vi "LoadInterfSetup.vi"(7 "BaseDataPath":path, 8 "ErrIn (NoErr)":errorcluster caption="entrée d'erreur (pas d'erreur)", 9 "IncrSession":bool=TRUE, 10 "LoadIntf?":bool=TRUE, 11 "Interface":path) -> (0 "error out":errorcluster caption="sortie d'erreur", 1 "Experiment Path":path, 2 "Session":i32, 3 "Interface en sortie":refnum<class "Interface.lvclass"> caption="DNL_LabVIEW Object out")   [LabVIEW 2012, in "Interface.lvclass"]
uses:
  Interface.lvclass
  Interface.lvclass/Interface.ctl
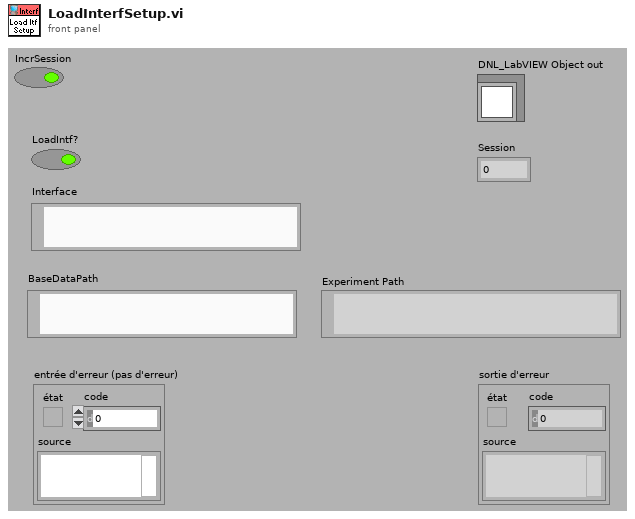
[diagram p1: front panel]
types:
  T1 = typedef "Interface.lvclass/CurveSetup.ctl" = cluster{"CurveName":string, "YParam":string, "XParam":string, "ZParam ":string, "GroupName":string, "LinWdth":u8, "PntCol":u32, "LinCol":u32, "LablFor":u8, "XScale":u32, "YScale":u32, "Interpol":u8, "DisplayName":string, "FillType":i16, "LineStyle":u8, "PntStyle":u8, "BarTyp":u8, "GraphIndex":i32, "Visible":bool, "XScaleName":string, "YScaleName":string, "XYGraph_Ref":refnum<vi>, "Data Only":bool, "DataQ Ref":refnum<queue>, "XParQ Ref":refnum<queue>, "XParamInd":i32, "ScanInd":i32}
  T2 = typedef "2DGraphSetup.ctl" = cluster{"ZDataIndex":i32, "XParIndex":i32, "YParIndex":i32, "FillLineFirst":bool}
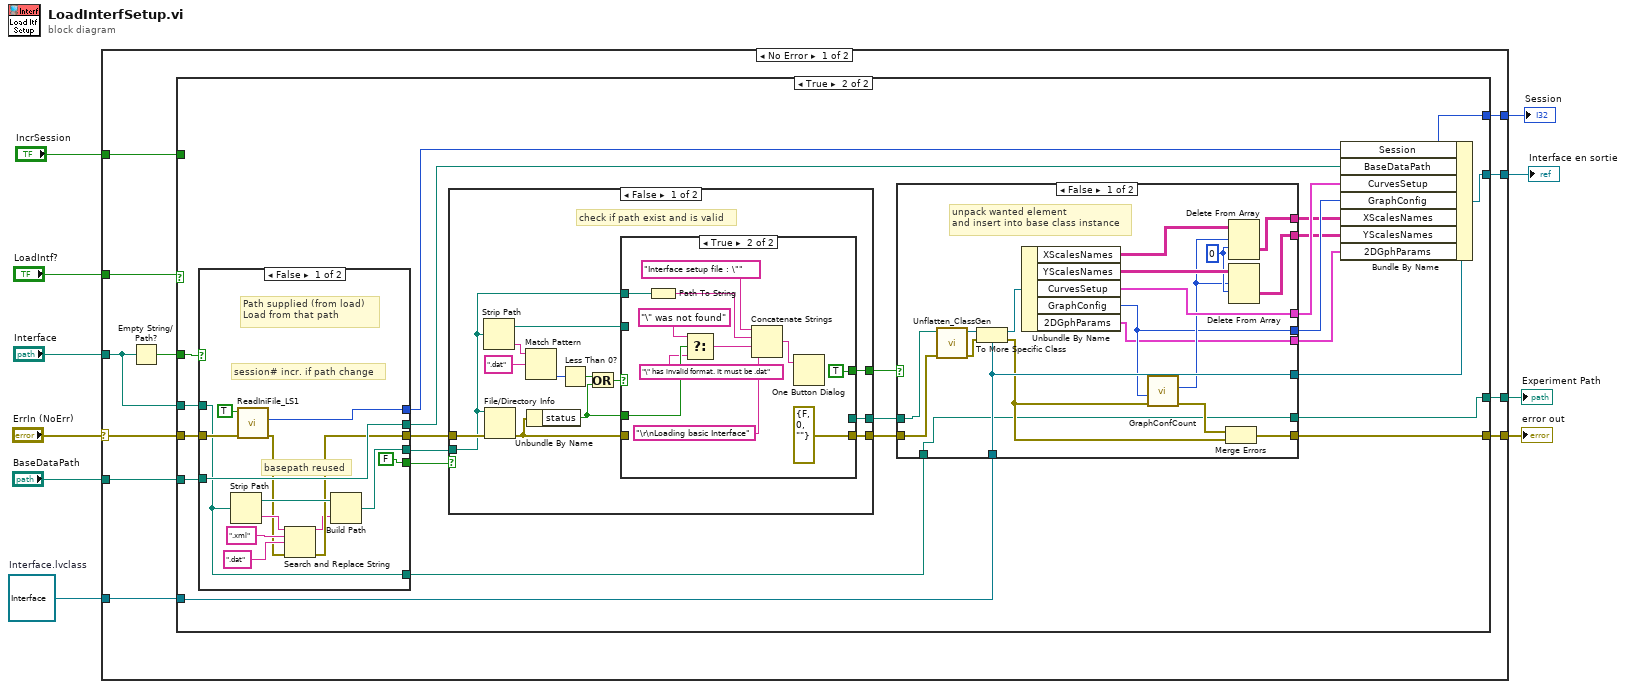
[diagram p0: block diagram]
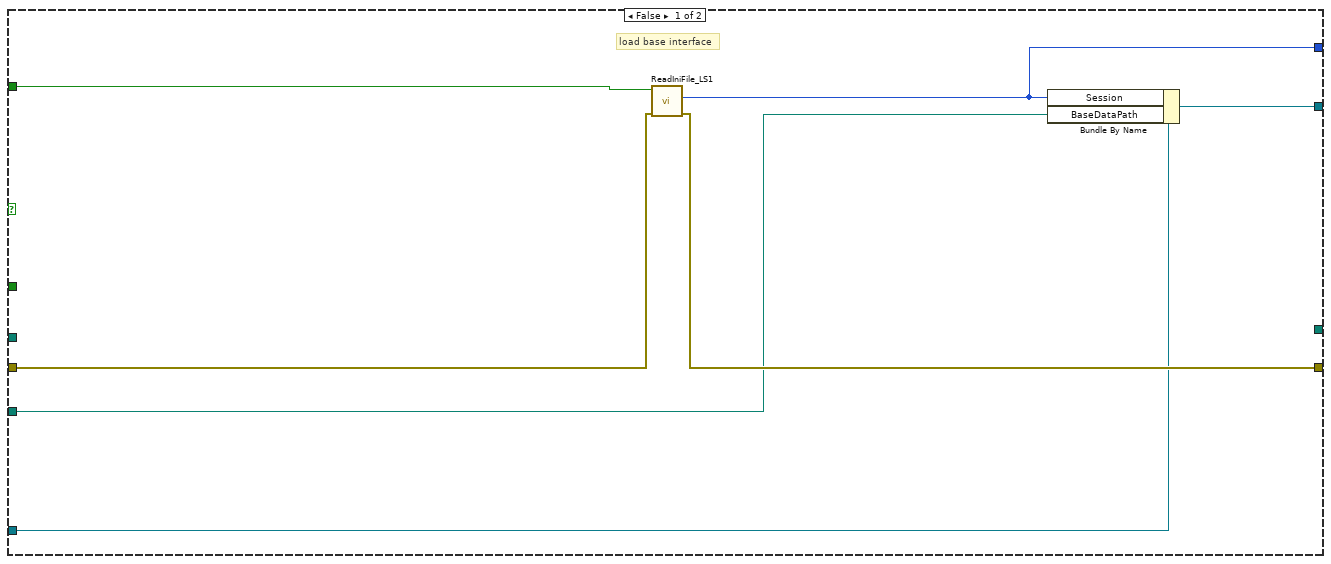
[diagram p2: hidden frame]
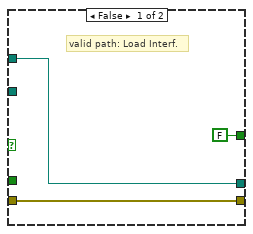
[diagram p3: hidden frame]
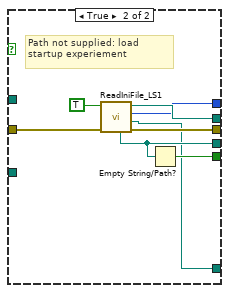
[diagram p5: hidden frame]
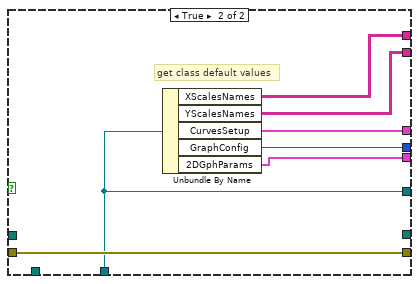
[diagram p6: hidden frame]
diagram:
  w4 = refnum<class "Interface.lvclass"> refnum  # Interface.lvclass
  n1 = case shown="No Error" "ErrIn (NoErr)" {
    selector: "ErrIn (NoErr)" -> [w20 w131]
    tunnel: [w19 w131] -> w9
    tunnel: [w18 w130] -> w8
    tunnel: w4 -> [w21 w130]
    tunnel: "LoadIntf?" -> [w17 _]
    tunnel: "Interface" -> [w15 _]
    tunnel: "BaseDataPath" -> [w14 _]
    tunnel: [w13 _] -> w3
    tunnel: "IncrSession" -> [w12 _]
    tunnel: [w11 _] -> w1
    frame No Error {
      n2 = Empty String/Path?(string/path=w15) -> (empty?=w16:bool)
      n3 = case shown="True" w17 {
        tunnel: w21 -> [w26 w38]
        tunnel: w20 -> [w28 w50]
        tunnel: [w27 w49] -> w19
        tunnel: [w25 w51] -> w18
        tunnel: w16 -> [_ w48]
        tunnel: w15 -> [_ w44]
        tunnel: w14 -> [w24 w39]
        tunnel: [w23 w31] -> w13
        tunnel: w12 -> [w22 _]
        tunnel: [_ w30] -> w11
        frame False {
          # "load base interface"
          n4 = call "ReadIniFile_LS1.vi"("Error in"=w28, "UpdateSess"=w22) -> ("Error out"=w27:errorcluster, "Session"=w23:i32)  [unwired: 4 in, 4 out]
          n5 = Bundle By Name(cluster=w26, "Session"=w23, "BaseDataPath"=w24) -> (w25:refnum<class "Interface.lvclass">)
        }
        frame True {
          n6 = case shown="False" w48 {
            tunnel: w50 -> [w94 w103]
            tunnel: [w91 w102] -> w40
            tunnel: [w92 w101] -> w31
            tunnel: [w84 w100] -> w45
            tunnel: [w82 w97] -> w46
            tunnel: [FALSE w99] -> w47
            tunnel: w44 -> [w90 _]
            tunnel: w39 -> [w91 _]
            tunnel: [w90 w96] -> w29
            frame False {
              # "basepath reused"
              # "session# incr. if path change"
              # "Path supplied (from load)\nLoad from that path"
              n7 = Strip Path(path=w90) -> (stripped path=w89:path, name=w88:string)
              n8 = call "ReadIniFile_LS1.vi"("Error in"=w94, "UpdateSess"=TRUE ("IncrSession")) -> ("Error out"=w85:errorcluster, "Session"=w92:i32)  [unwired: 4 in, 4 out]
              n9 = Search and Replace String(input string=w88, search string=".xml", replace string=".dat" ("replace string (\"\")"), error in=w85) -> (result string=w83:string, error out=w84:errorcluster)  [unwired: 4 in, 2 out]
              n10 = Build Path(base path=w89, name or relative path=w83) -> (appended path=w82:path)
            }
            frame True {
              # "Path not supplied: load startup experiement"
              n11 = call "ReadIniFile_LS1.vi"("Error in"=w103, "UpdateSess"=TRUE ("IncrSession")) -> ("Error out"=w100:errorcluster, "Experiment"=w96:path, "Session"=w101:i32, "BaseDataPath"=w102:path, "Interface"=w97:path)  [unwired: 4 in, 1 out]
              n12 = Empty String/Path?(string/path=w97) -> (empty?=w99:bool)
            }
          }
          n13 = case shown="False" w47 {
            selector: w47 -> [_ w79]
            tunnel: [w57 w81] -> w42
            tunnel: w45 -> [w63 w81]
            tunnel: w46 -> [w58 w80]
            tunnel: [w59 w80] -> w41
            tunnel: [w54 w79] -> w43
            frame False {
              # "check if path exist and is valid"
              n14 = Strip Path(path=w58) -> (stripped path=w53:path, name=w52:string)
              n15 = File/Directory Info(path=w58, error in=w63) -> (error out=w56:errorcluster)  [unwired: 6 out]
              n16 = Match Pattern(string=w52, regular expression=".dat" ("expression régulière")) -> (offset past match=w61:i32)  [unwired: 1 in, 3 out]
              n17 = Unbundle By Name(w56) -> ("status"=w55:bool)
              n18 = Less Than 0?(x=w61) -> (x < 0?=w62:bool)
              n19 = Or(x=w62, y=w55) -> (x .or. y?=w60:bool)
              n20 = case shown="True" w60 {
                tunnel: [w67 _] -> w59
                tunnel: w58 -> [w67 w77]
                tunnel: [w66 errorcluster {"status"=FALSE, "code"=0, "source"=""} ("error out")] -> w57
                tunnel: w56 -> [w66 _]
                tunnel: w55 -> [_ w76]
                tunnel: [FALSE ("true") TRUE ("true")] -> w54
                tunnel: w53 -> [_ _]
                frame False {
                  # "valid path: Load Interf."
                }
                frame True {
                  n21 = Path To String(path=w77) -> (string=w72:string)
                  n22 = Select(t="\" was not found" ("message"), s=w76, f="\" has invalid format. It must be .dat" ("message")) -> (s? t:f=w73:string)
                  n23 = Concatenate Strings("Interface setup file : \"" ("message"), w72, w73, "\r\nLoading basic Interface" ("message")) -> (w71:string)
                  n24 = One Button Dialog(message=w71) -> ()  [unwired: 1 in, 1 out]
                }
              }
            }
            frame True {
              # "empty startup path"
            }
          }
          n25 = case shown="False" w43 {
            tunnel: [w116 w129] -> w49
            tunnel: w42 -> [w122 w129]
            tunnel: w41 -> [w105 _]
            tunnel: w38 -> [w119 w126]
            tunnel: [w119 w126] -> w37
            tunnel: [w117 w128] -> w36
            tunnel: [w107 w127] -> w35
            tunnel: [w114 w124] -> w34
            tunnel: [w111 w125] -> w33
            tunnel: [w106 w123] -> w32
            tunnel: [w104 _] -> w30
            tunnel: w29 -> [w104 _]
            frame False {
              w112 = 0 ("indice (ligne)")
              # "unpack wanted element\nand insert into base class instance"
              n26 = call <userlib>:"Unflatten_ClassGen.vi"("error in (no error)"=w122, "XML File Path"=w105) -> ("sortie d'erreur"=w120:errorcluster, "LabVIEW Object"=w121:refnum<class>)  [unwired: 8 in]
              n27 = To More Specific Class(target class=w119, reference=w121, error in=w120) -> (specific class reference=w118:refnum<class "Interface.lvclass">, error out=w110:errorcluster)
              n28 = Unbundle By Name(w118) -> ("XScalesNames"=w115:string[][], "YScalesNames"=w113:string[][], "CurvesSetup"=w117:T1[], "GraphConfig"=w107:i32, "2DGphParams"=w106:T2[])
              n29 = call "GraphConfCount.vi"("error in (no error)"=w110, "Configuration"=w107) -> ("error out"=w108:errorcluster, "GraphCount"=w109:i32)  [unwired: 8 in]
              n30 = Merge Errors(w108, w110) -> (w116:errorcluster)
              n31 = Delete From Array(array=w115, length=w109, index (row)=w112) -> (deleted portion=w114:string[][])  [unwired: 1 in, 1 out]
              n32 = Delete From Array(array=w113, length=w109, index (row)=w112) -> (deleted portion=w111:string[][])  [unwired: 1 in, 1 out]
            }
            frame True {
              # "get class default values"
              n33 = Unbundle By Name(w126) -> ("XScalesNames"=w124:string[][], "YScalesNames"=w125:string[][], "CurvesSetup"=w128:T1[], "GraphConfig"=w127:i32, "2DGphParams"=w123:T2[])
            }
          }
          n34 = Bundle By Name(cluster=w37, "Session"=w31, "BaseDataPath"=w40, "CurvesSetup"=w36, "GraphConfig"=w35, "XScalesNames"=w34, "YScalesNames"=w33, "2DGphParams"=w32) -> (w51:refnum<class "Interface.lvclass">)
        }
      }
    }
    frame Error {
    }
  }
  "error out" <- w9
  "Interface en sortie" <- w8
  "Session" <- w3
  "Experiment Path" <- w1
